vi "Sys config window-Set disabled states-retd.vi"(8 "error in (no error)":errorcluster) -> (0 "error out":errorcluster)   [LabVIEW 2020]
uses:
  Globals/Sys Config window globals.vi
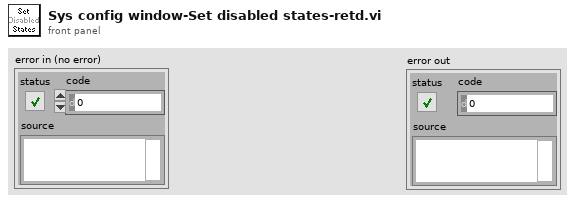
[diagram p1: front panel]
types:
  T1 = enum8{"Enabled", "Disabled", "Disabled and Grayed Out"}
  T2 = typedef "HW config window refs cluster.ctl" = cluster{"VI's reference":refnum<vi>, "menu reference":refnum<k9>, "Pane":refnum<vi>, "Config Tab Control":refnum<vi>, "Triggers sub-tab control":refnum<vi>, "Microscope ID":refnum<vi>, "Microscope Type":refnum<vi>, "Revision Number":refnum<vi>, "Advanced Imaging":refnum<vi>, "Max Allowed Trial Length":refnum<vi>, "Initial Scan Resolution":refnum<vi>, "Initial Acceptance Angle":refnum<vi>, "Initial Laser Wavelength [nm] ":refnum<vi>, "Initial Dwell Time [us]":refnum<vi>, "Error Logging":refnum<vi>, "Performance Monitoring":refnum<vi>, "Ctrl FPGA available":refnum<vi>, "Control HW config":refnum<vi>, "Control System Config":refnum<vi>, "General trigger settings":refnum<vi>, "Trigger HW config":refnum<vi>, "Externalise Triggers":refnum<vi>, "[Triggers output setup]":refnum<vi>, "DAQ FPGA HW Config":refnum<vi>, "DAQ FPGA System Config":refnum<vi>, "Pockels AO":refnum<vi>, "Hard shutter AO":refnum<vi>, "PMT AOs":refnum<vi>, "Galvo AO":refnum<vi>, "Power meter AI":refnum<vi>, "XY stage available":refnum<vi>, "XY Stage config cluster":refnum<vi>, "Z stage available":refnum<vi>, "Z Stage config cluster":refnum<vi>, "Encoder available":refnum<vi>, "Encoder":refnum<vi>, "Encoder IP address":refnum<vi>, "Encoder port":refnum<vi>, "Wheel radius (cm)":refnum<vi>, "Demo mode":refnum<vi>, "Swap XY on stage":refnum<vi>, "Number of AODs":refnum<vi>, "Axial MC Supported":refnum<vi>, "MC Supported":refnum<vi>, "Computer MAC add.":refnum<vi>, "Cam VidRec available":refnum<vi>, "Cam VidRec":refnum<vi>, "DO flag-Video record":refnum<vi>, "DO flag-Trial start":refnum<vi>, "AOD Settings (distilled)":refnum<vi>, "Pockels cal.Dwell time (µs)":refnum<vi>, "Pockels cal.Zoom":refnum<vi>, "Current Objective":refnum<vi>, "[Obj. Calib. Settings]":refnum<vi>, "Laser Wavelength":refnum<vi>, "Laser Power Control \nHW config":refnum<vi>, "Laser 1 available":refnum<vi>, "Laser 1 config":refnum<vi>, "Prechirper 1 available":refnum<vi>, "Prechirper 1 config":refnum<vi>, "PreChirp Preset Values":refnum<vi>, "[PreChirper Preset \nCalibration Values]":refnum<vi>, "Prechirper Constants":refnum<vi>}
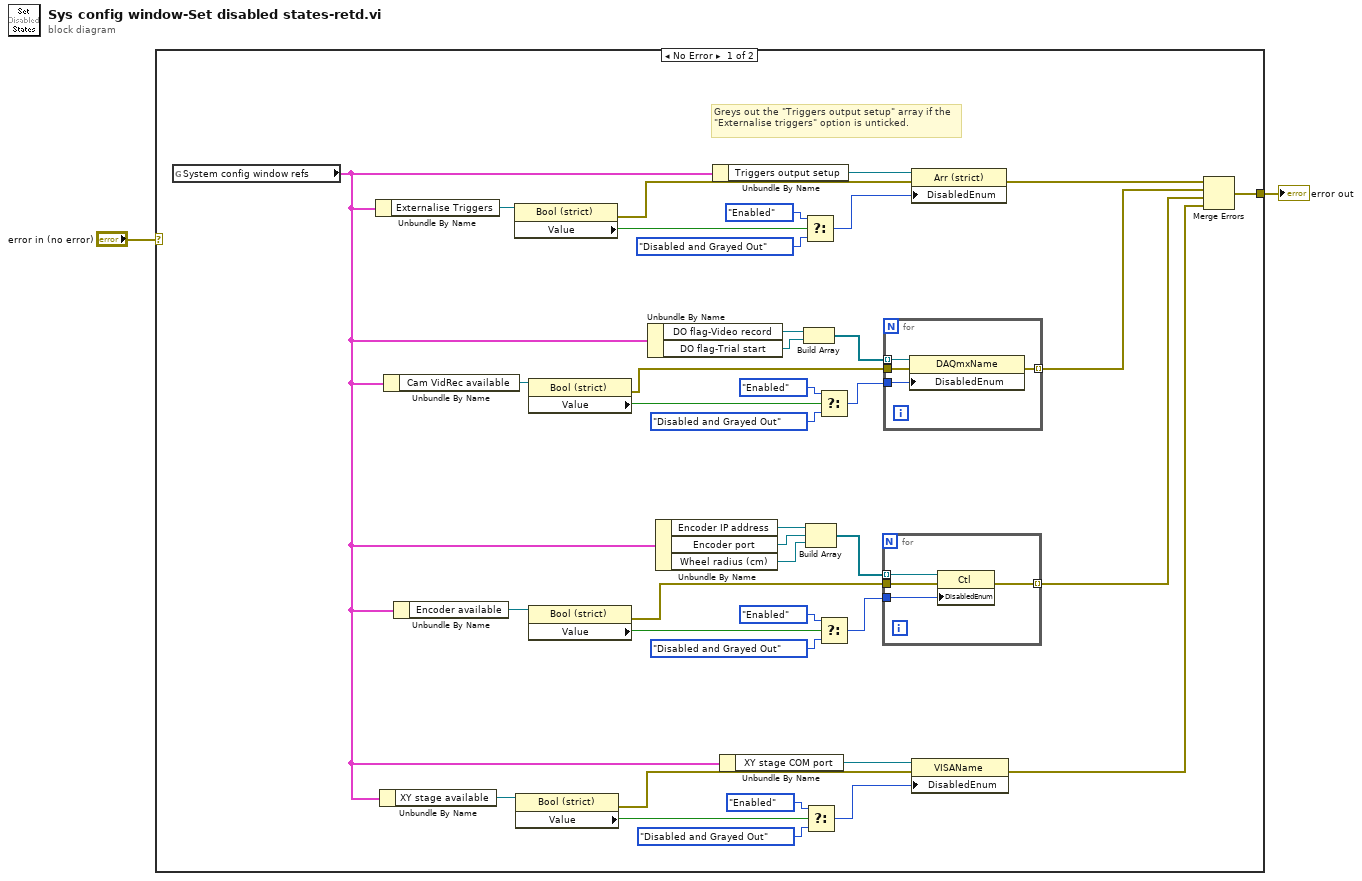
[diagram p0: block diagram]
diagram:
  n1 = case shown="No Error" "error in (no error)" {
    selector: "error in (no error)" -> [_ w50]
    tunnel: [w27 w50] -> w2
    frame No Error {
      # "Greys out the \"Triggers output setup\" array if the \"Externalise triggers\" option is unticked."
      n2 = global read "Sys Config window globals.vi" "System config window refs"() -> (w14:T2)
      n3 = Unbundle By Name(w14) -> ("Externalise Triggers"=w41:refnum<vi>)
      n4 = Unbundle By Name(w14) -> ("XY stage available"=w15:refnum<vi>)
      n5 = Unbundle By Name(w14) -> ("Cam VidRec available"=w31:refnum<vi>)
      n6 = Unbundle By Name(w14) -> ("Encoder available"=w26:refnum<vi>)
      n7 = property class="Bool (strict)"(reference=w41) -> (error out=w35:errorcluster, "Value"=w39:bool)  [unwired: 1 in, 1 out]
      n8 = property class="Bool (strict)"(reference=w15) -> (error out=w21:errorcluster, "Value"=w17:bool)  [unwired: 1 in, 1 out]
      n9 = property class="Bool (strict)"(reference=w31) -> (error out=w22:errorcluster, "Value"=w32:bool)  [unwired: 1 in, 1 out]
      n10 = property class="Bool (strict)"(reference=w26) -> (error out=w4:errorcluster, "Value"=w25:bool)  [unwired: 1 in, 1 out]
      n11 = Unbundle By Name(w14) -> ("DO flag-Video record"=w11:refnum<vi>, "DO flag-Trial start"=w12:refnum<vi>)
      n12 = Unbundle By Name(w14) -> ("Encoder IP address"=w9:refnum<vi>, "Encoder port"=w8:refnum<vi>, "Wheel radius (cm)"=w3:refnum<vi>)
      n13 = Unbundle By Name(w14) -> ("Triggers output setup"=w40:refnum<vi>)
      n14 = Unbundle By Name(w14) -> ("XY stage COM port"=w16:refnum<vi>)
      n15 = Build Array(w11, w12) -> (w10:refnum<vi>[])
      n16 = Select(t=T1."Enabled" ("Disabled"), s=w39, f=T1."Disabled and Grayed Out" ("Disabled")) -> (s? t:f=w36:T1)
      n17 = Build Array(w9, w8, w3) -> (w7:refnum<vi>[])
      n18 = Select(t=T1."Enabled" ("Disabled"), s=w17, f=T1."Disabled and Grayed Out" ("Disabled")) -> (s? t:f=w20:T1)
      n19 = Select(t=T1."Enabled" ("Disabled"), s=w32, f=T1."Disabled and Grayed Out" ("Disabled")) -> (s? t:f=w29:T1)
      n20 = Select(t=T1."Enabled" ("Disabled"), s=w25, f=T1."Disabled and Grayed Out" ("Disabled")) -> (s? t:f=w6:T1)
      n21 = for {
        tunnel: [w45] -> w5 mode=indexing
        tunnel: w6 -> [w44]
        tunnel: w4 -> [w43]
        tunnel: w7 -> [w42] mode=indexing
        n22 = property class="Ctl"(reference=w42, error in=w43, "DisabledEnum"=w44) -> (error out=w45:errorcluster)  [unwired: 1 out]
      }
      n23 = for {
        tunnel: [w49] -> w30 mode=indexing
        tunnel: w29 -> [w48]
        tunnel: w22 -> [w47]
        tunnel: w10 -> [w46] mode=indexing
        n24 = property class="DAQmxName"(reference=w46, error in=w47, "DisabledEnum"=w48) -> (error out=w49:errorcluster)  [unwired: 1 out]
      }
      n25 = property class="Arr (strict)"(reference=w40, error in=w35, "DisabledEnum"=w36) -> (error out=w28:errorcluster)  [unwired: 1 out]
      n26 = property class="VISAName"(reference=w16, error in=w21, "DisabledEnum"=w20) -> (error out=w13:errorcluster)  [unwired: 1 out]
      n27 = Merge Errors(w28, w30, w5, w13) -> (w27:errorcluster)
    }
    frame Error {
    }
  }
  "error out" <- w2
